vi "CSM - Filter Duplicated Lines.vi"(1 "Keep First Matched? (T)":bool=TRUE, 5 "States In":string, 7 "Option":enum16{"State", "No Comments", "Line"}(ring)) -> (6 "States Out":string)   [LabVIEW 2017, in "Communicable State Machine.lvlib"]
doc: "Filters duplicated lines in the CSM state queue.\n\n\n> [!NOTE] <b>CSM State Queue Operation API</b>\n>\n> This type of API only concatenates message strings and does not send messages directly. The message is sent and the operation executed within the Parse State Queue++ VI. Unlike the Message Building API, this type of API includes a CSM state queue string input, which is equivalent to inserting a message into the state queue.\n\n\n-- <b>Controls</b> --\n- <b>Keep First Matched? (T)</b>: Whether to keep the first matched item. The default is TRUE.\n- <b>States In</b>: The entire state description string to filter.\n- <b>Option</b>: Filter option.\n\n-- <b>Indicators</b> --\n- <b>States Out</b>: The filtered state description string."
uses:
  Communicable State Machine.lvlib
  _Shared/CSM Shared.lvlib
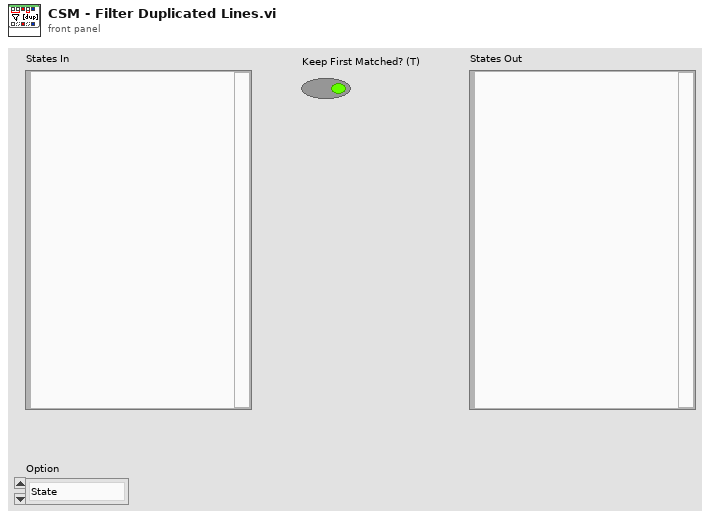
[diagram p1: front panel]
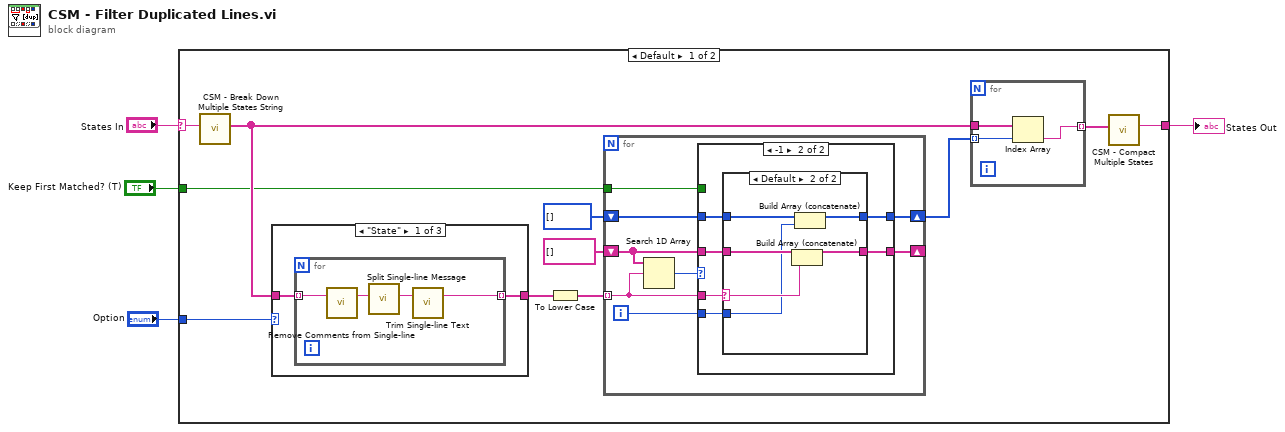
[diagram p0: block diagram]
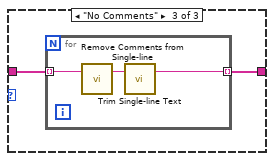
[diagram p3: hidden frame]
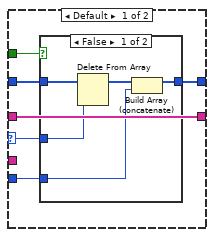
[diagram p4: hidden frame]
diagram:
  n1 = case shown="Default" "States In" {
    selector: "States In" -> [w15 w65]
    tunnel: [w14 w65] -> w3
    tunnel: "Option" -> [w7 _]
    tunnel: "Keep First Matched? (T)" -> [w5 _]
    frame Default {
      n2 = call "CSM - Break Down Multiple States String.vi"("States"=w15) -> ("Multiple States"=w13:string[])  [unwired: 10 in]
      n3 = case shown="\"State\"" w7 {
        tunnel: w13 -> [w17 w22 w24]
        tunnel: [w16 w22 w23] -> w11
        frame "State" {
          n4 = for {
            tunnel: w17 -> [w20] mode=indexing
            tunnel: [w18] -> w16 mode=indexing
            n5 = call "Remove Comments from Single-line.vi"("single-line text"=w20) -> ("single-line text without comments"=w21:string)  [unwired: 2 in]
            n6 = call "Split Single-line Message.vi"("single-line text"=w21) -> ("state"=w19:string)  [unwired: 6 in, 3 out]
            n7 = call "Trim Single-line Text.vi"("single-line text"=w19) -> ("trimed text"=w18:string)  [unwired: 2 in]
          }
        }
        frame "Line" {
        }
        frame "No Comments" {
          n8 = for {
            tunnel: w24 -> [w26] mode=indexing
            tunnel: [w25] -> w23 mode=indexing
            n9 = call "Remove Comments from Single-line.vi"("single-line text"=w26) -> ("single-line text without comments"=w27:string)  [unwired: 2 in]
            n10 = call "Trim Single-line Text.vi"("single-line text"=w27) -> ("trimed text"=w25:string)  [unwired: 2 in]
          }
        }
      }
      n11 = To Lower Case(string=w11) -> (all lower case string=w6:string[])
      n12 = for {
        tunnel: w6 -> [w37] mode=indexing
        shift-right: [w36] -> _
        shift-left: string[] [] -> [w35]
        shift-right: [w33] -> w8
        shift-left: i32[] [] -> [w32]
        tunnel: w5 -> [w31]
        i -> [w34]
        n13 = Search 1D Array(1D array=w35, element=w37) -> (index of element=w38:i32)  [unwired: 1 in]
        n14 = case shown="-1" w38 {
          selector: w38 -> [w42 _]
          tunnel: w37 -> [_ w56]
          tunnel: [w44 w54] -> w36
          tunnel: w35 -> [w44 w55]
          tunnel: w34 -> [w40 w51]
          tunnel: [w41 w52] -> w33
          tunnel: w32 -> [w43 w53]
          tunnel: w31 -> [w39 _]
          frame Default {
            n15 = case shown="False" w39 {
              tunnel: w43 -> [w49 w50]
              tunnel: w42 -> [w47 _]
              tunnel: [w46 w50] -> w41
              tunnel: w40 -> [w45 _]
              frame False {
                n16 = Delete From Array(array=w49, index=w47) -> (array with subset deleted=w48:i32[])  [unwired: 1 in, 1 out]
                n17 = Build Array (concatenate)(w48, w45) -> (w46:i32[])
              }
              frame True {
              }
            }
          }
          frame -1 {
            n18 = case shown="Default" w56 {
              selector: w56 -> [_ w64]
              tunnel: w55 -> [w57 w63]
              tunnel: [w57 w62] -> w54
              tunnel: w53 -> [w58 w61]
              tunnel: [w58 w60] -> w52
              tunnel: w51 -> [_ w59]
              frame "" {
              }
              frame Default {
                n19 = Build Array (concatenate)(w63, w64) -> (w62:string[])
                n20 = Build Array (concatenate)(w61, w59) -> (w60:i32[])
              }
            }
          }
        }
      }
      n21 = for {
        tunnel: w8 -> [w30] mode=indexing
        tunnel: w13 -> [w29]
        tunnel: [w28] -> w12 mode=indexing
        n22 = Index Array(array=w29, index=w30) -> (element=w28:string)
      }
      n23 = call "CSM - Compact Multiple States.vi"("Multiple States"=w12) -> ("States"=w14:string)  [unwired: 9 in]
    }
    frame "" {
    }
  }
  "States Out" <- w3
